vi "Sending_TestMode_Recipe_Sub_VI_Sample.vi"(0 "Socket IP Address":string="192.168.1.100", 1 "Socket Port Numeber":u16=1600, 2 "Receipe Msg ID":i32, 3 "Receipe Message length":i32, 4 "TestAmplitudeLoopC1":i32, 5 "TestAmplitudeLoopC2":i32, 6 "TestPhaseLoopI":i32, 7 "TestPhaseLoopCF":i32, 8 "TestFrequencyHigh":i32, 9 "TestFrequencyLow":i32, 10 "TestAmplitude":i32, 13 "error in (no error)":errorcluster, 14 "Response ID":u8=66) -> (15 "connection ID":refnum<k5>, 17 "error out":errorcluster)   [LabVIEW 2017]
panel:
  out "rest of the binary string":string
  out "*(type *) &x 2":u8
  out "*(type *) &x":u8
  out "String":string=" Success"
  out "bytes written 2":i32
  # "Please find the below information,\n                               \n                                                                Default                 Min                        Max                                                                                         \n \n20KHz System:\n-------------------\nSeekFreqLimitLow                           195000                  195000                     -\nSeekFreqLimitHigh                          205000                       -                         205000\n \n30KHz System:\n-------------------\nSeekFreqLimitLow                           292500                  292500                     -\nSeekFreqLimitHigh                          307500                       -                         307500\n \n40KHz System:\n-------------------\nSeekFreqLimitLow                           395000                  390000                     -\nSeekFreqLimitHigh                          405000                       -                         410000"
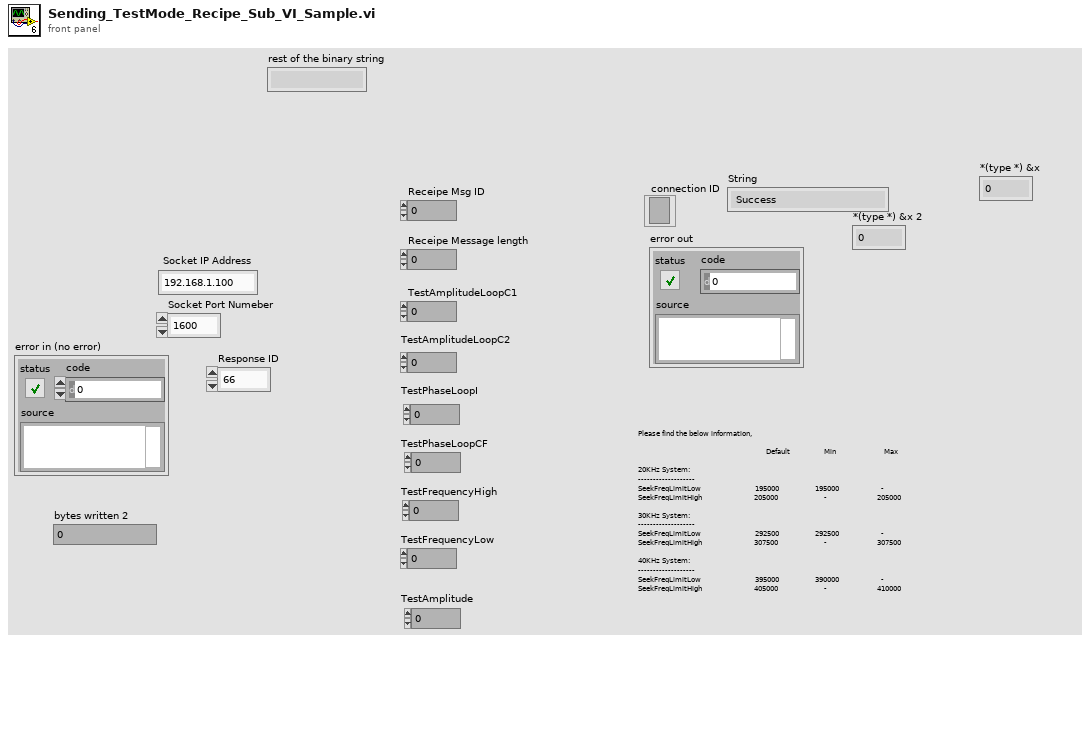
[diagram p1: front panel]
types:
  T1 = enum16{"big-endian, network order", "native, host order", "little-endian"}
  T2 = cluster{"TestAmplitude":i32, "TestFrequencyLow":i32, "TestFrequencyHigh":i32, "TestPhaseLoopCF":i32, "TestPhaseLoopI":i32, "TestAmplitudeLoopC2":i32, "TestAmplitudeLoopC1":i32, "Receipe Message length":i32, "Receipe Msg ID":i32}
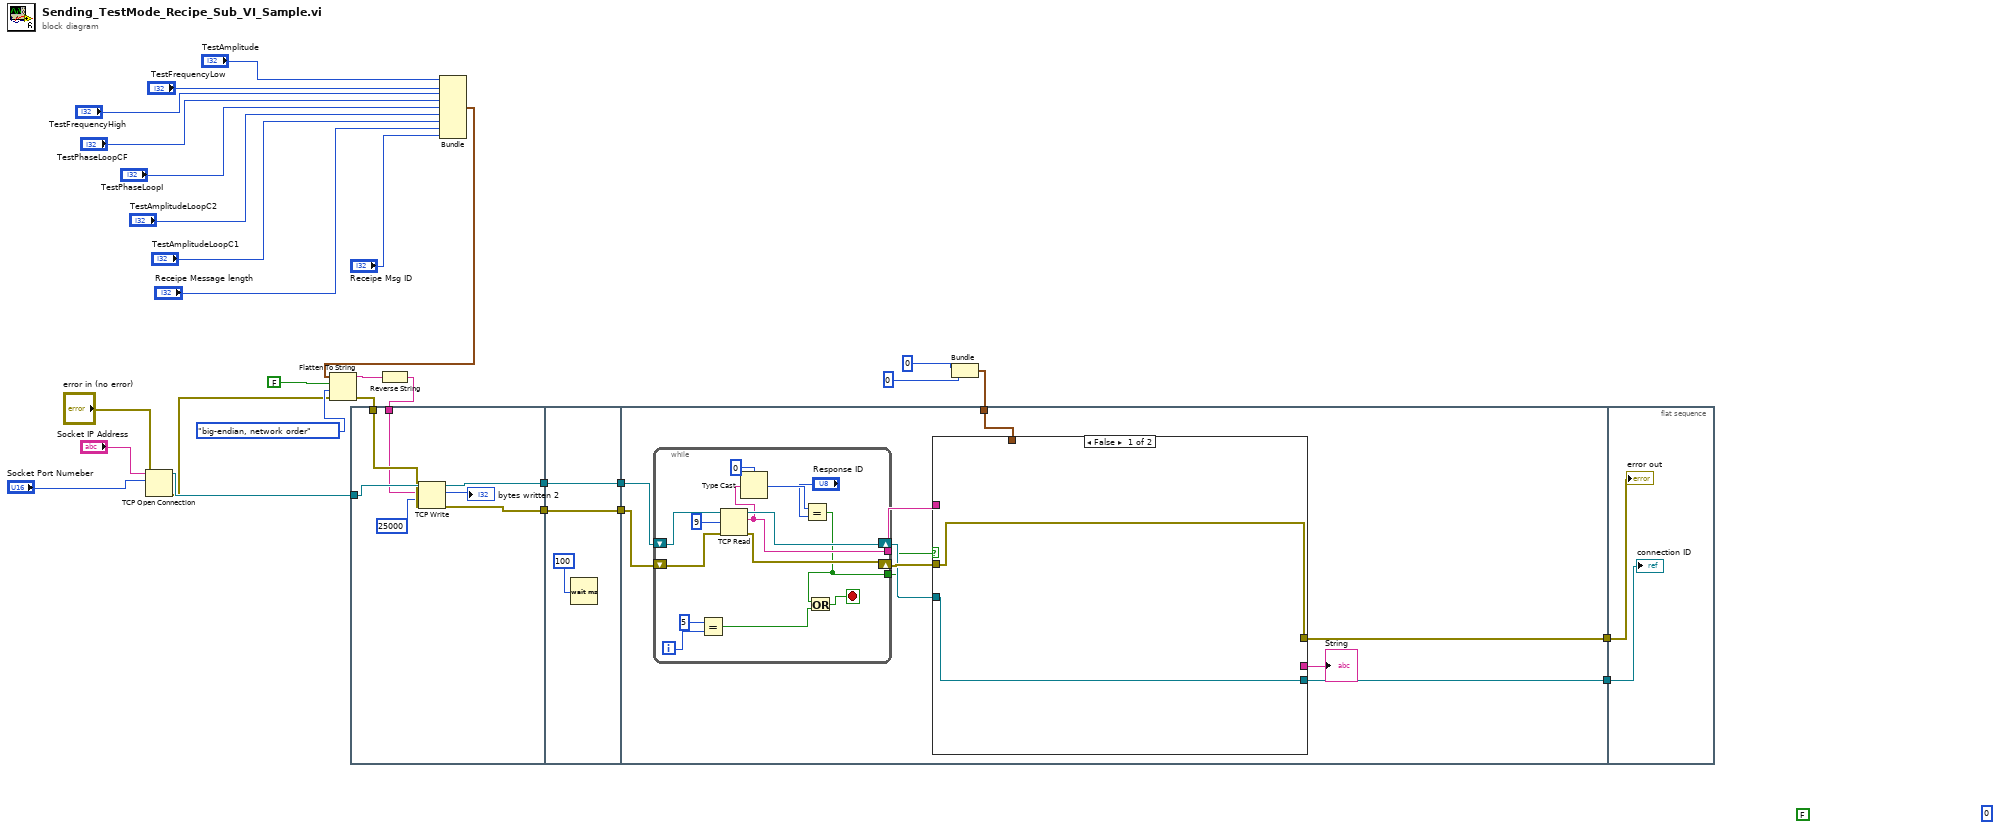
[diagram p0: block diagram]
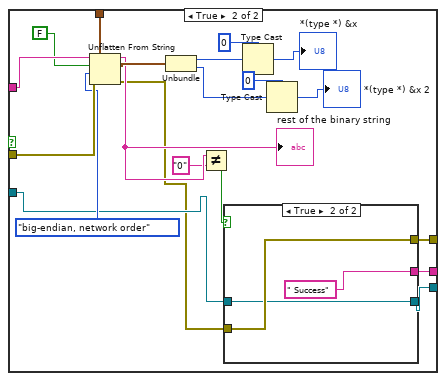
[diagram p2: hidden frame]
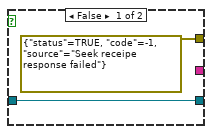
[diagram p3: hidden frame]
diagram:
  (unwired) u8 0
  (unwired) FALSE ("data includes array or string size? (T)")
  n1 = TCP Open Connection(address="Socket IP Address", remote port or service name="Socket Port Numeber", error in (no error)="error in (no error)") -> (connection ID=w21:refnum<k5>, error out=w20:errorcluster)  [unwired: 2 in]
  n2 = flat-sequence {
    tunnel: w21 -> [w34]
    tunnel: w19 -> [w33]
    tunnel: w17 -> [w32]
    tunnel: [w36] -> w29
    tunnel: [w35] -> w28
    tunnel: w29 -> [w39]
    tunnel: w28 -> [w38]
    tunnel: [w39] -> w27
    tunnel: [w38] -> w26
    tunnel: w27 -> [w49]
    tunnel: w26 -> [w48]
    tunnel: w4 -> [w43]
    tunnel: [w42] -> w2
    tunnel: [w41] -> w1
    tunnel: w2 -> [w92]
    tunnel: w1 -> [w91]
    frame #0 {
      n3 = TCP Write(connection ID=w34, data in=w32, error in (no error)=w33, 9:25000 ("timeout ms (25000)")) -> (connection ID out=w36:refnum<k5>, bytes written=→"bytes written 2":i32, error out=w35:errorcluster)
    }
    frame #1 {
      n4 = Wait (ms)(milliseconds to wait=u32 100) -> ()  [unwired: 1 out]
    }
    frame #2 {
      n5 = while {
        tunnel: [w86] -> w46
        shift-right: [w88] -> w45
        shift-left: w49 -> [w90]
        shift-right: [w82] -> w47
        shift-left: w48 -> [w89]
        tunnel: [w80] -> w44
        i -> [w79]
        stop <- w81 stop-if-true
        n6 = Equal?(x=5, y=w79) -> (x = y?=w77:bool)
        n7 = TCP Read(connection ID=w90, bytes to read=9, error in (no error)=w89) -> (connection ID out=w88:refnum<k5>, data out=w86:string, error out=w82:errorcluster)  [unwired: 2 in]
        n8 = Type Cast(type=u8 0, x=w86) -> (*(type *) &x=w84:u8)
        n9 = Equal?(x=w84, y="Response ID") -> (x = y?=w80:bool)
        n10 = Or(x=w80, y=w77) -> (x .or. y?=w81:bool)
      }
      n11 = case shown="False" w44 {
        tunnel: w47 -> [w50 w71]
        tunnel: w46 -> [_ w70]
        tunnel: w45 -> [w51 w62]
        tunnel: w43 -> [_ w66]
        tunnel: [w51 w61] -> w42
        tunnel: [w50 w60] -> w41
        tunnel: [_ w59] -> w40
        frame False {
        }
        frame True {
          n12 = Unflatten From String(type=w66, binary string=w70, data includes array or string size? (T)=FALSE, byte order (0:big-endian, network order)=T1."big-endian, network order", error in (no error)=w71) -> (rest of the binary string=w65:string, value=w67:cluster{i32, i32}, error out=w58:errorcluster)
          "rest of the binary string" <- w65
          n13 = Unbundle(w67) -> (w57:i32, w52:i32)
          n14 = Not Equal?(x=w65, y="0") -> (x != y?=w63:bool)
          n15 = case shown="True" w63 {
            tunnel: [errorcluster {"status"=TRUE, "code"=-1, "source"="Seek receipe response failed"} ("error constant") w75] -> w60
            tunnel: w62 -> [w72 w74]
            tunnel: [w72 w74] -> w61
            tunnel: [_ " Success"] -> w59
            tunnel: w58 -> [_ w75]
            frame False {
            }
            frame True {
            }
          }
          n16 = Type Cast(type=u8 0, x=w57) -> (*(type *) &x=→"*(type *) &x":u8)
          n17 = Type Cast(type=u8 0, x=w52) -> (*(type *) &x=→"*(type *) &x 2":u8)
        }
      }
      "String" <- w40
    }
    frame #3 {
      "connection ID" <- w92
      "error out" <- w91
    }
  }
  n18 = Bundle("TestAmplitude"="TestAmplitude", "TestFrequencyLow"="TestFrequencyLow", "TestFrequencyHigh"="TestFrequencyHigh", "TestPhaseLoopCF"="TestPhaseLoopCF", "TestPhaseLoopI"="TestPhaseLoopI", "TestAmplitudeLoopC2"="TestAmplitudeLoopC2", "TestAmplitudeLoopC1"="TestAmplitudeLoopC1", "Receipe Message length"="Receipe Message length", "Receipe Msg ID"="Receipe Msg ID") -> (w7:T2)  [unwired: 1 in]
  n19 = Flatten To String(anything=w7, prepend array or string size? (T)=FALSE, byte order (0:big-endian, network order)=T1."big-endian, network order", error in (no error)=w20) -> (data string=w18:string, error out=w19:errorcluster)  [unwired: 1 out]
  n20 = Reverse String(1:w18) -> (0:w17:string)
  n21 = Bundle(0, 0) -> (w4:cluster{i32, i32})  [unwired: 1 in]
